vi "UpdateSupportedFunctions.vi"() -> ()   [LabVIEW 2014, in "Raspberry Pi Compatible Compiler for LabVIEW.lvlib" / "Python Functions.lvlib"]
uses:
  Python Functions.lvlib
panel:
  in  "supported functions VI":string="SupportedFunctions.vi"
  in  "package":path=path "E:/Work/RasPi/pyVI"
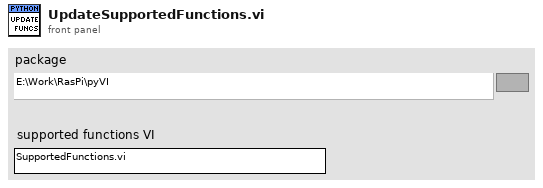
[diagram p1: front panel]
types:
  T1 = typedef "Raspberry Pi Compatible Compiler for LabVIEW.lvlib/Python Functions.lvlib/FunctionsTD.ctl" = cluster{"module":string, "short name":string, "docstrings":T2}[]
  T2 = typedef "Raspberry Pi Compatible Compiler for LabVIEW.lvlib/Python Functions.lvlib/DocstringTD.ctl" = cluster{"type":string, "name":string, "docstring":string}
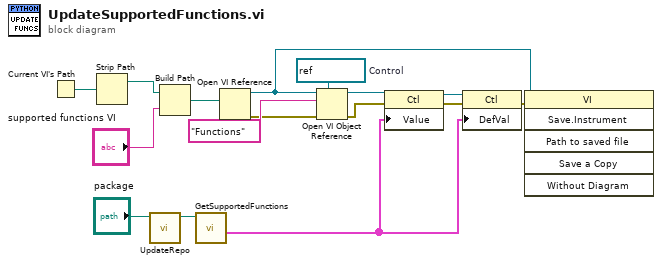
[diagram p0: block diagram]
diagram:
  w12 = refnum<vi> refnum  # Control
  n1 = Current VI's Path() -> (path=w4:path)
  n2 = Strip Path(path=w4) -> (stripped path=w3:path)  [unwired: 1 out]
  n3 = call "UpdateRepo.vi"("package"="package") -> ("package out"=w2:path)  [unwired: 10 in]
  n4 = Build Path(base path=w3, name or relative path="supported functions VI") -> (appended path=w15:path)
  n5 = call "GetSupportedFunctions.vi"("package"=w2) -> ("Functions"=w7:T1)  [unwired: 9 in, 1 out]
  n6 = Open VI Reference(vi path=w15) -> (vi reference=w5:refnum<vi>, error out=w13:errorcluster)  [unwired: 5 in]
  n7 = Open VI Object Reference(7:w12, 8:w13, 10:"Functions" ("Control Name"), 11:w5) -> (0:w10:errorcluster, 3:w11:refnum<vi>)
  n8 = property class="Ctl"(reference=w11, error in=w10, "Value"=w7) -> (reference out=w9:refnum<vi>, error out=w8:errorcluster)
  n9 = property class="Ctl"(reference=w9, error in=w8, "DefVal"=w7) -> (error out=w6:errorcluster)  [unwired: 1 out]
  n10 = invoke class="VI" method="Save.Instrument"(reference=w5, error in=w6) -> ()  [unwired: 4 in, 6 out]
